vi "registerEvents.vi"(8 "error in (no error)":errorcluster, 10 "registeredEvents":string[][](array[string]), 11 "tcpServer in":refnum<class "TcpServer.lvclass">) -> (0 "error out":errorcluster, 3 "tcpServer out":refnum<class "TcpServer.lvclass">)   [LabVIEW 2018, in "TcpServer.lvclass"]
doc: "Inform the TCP Server which events are registered and allowed to be processed."
uses:
  TcpServer.lvclass
  TcpServer.lvclass/TcpServer.ctl
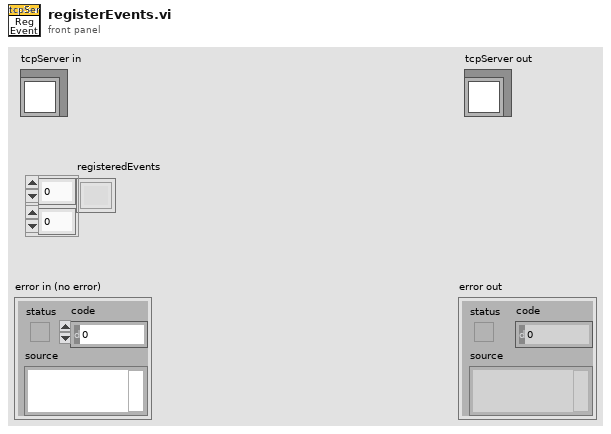
[diagram p1: front panel]
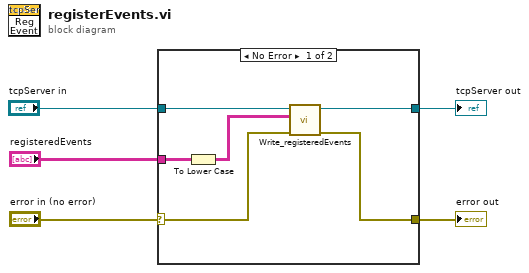
[diagram p0: block diagram]
diagram:
  n1 = case shown="No Error" "error in (no error)" {
    selector: "error in (no error)" -> [w8 w13]
    tunnel: [w7 w13] -> w4
    tunnel: [w10 w12] -> w2
    tunnel: "tcpServer in" -> [w11 w12]
    tunnel: "registeredEvents" -> [w9 _]
    frame No Error {
      n2 = To Lower Case(string=w9) -> (all lower case string=w6:string[][])
      n3 = call "Write_registeredEvents.vi"("error in (no error)"=w8, "registeredEvents"=w6, "TcpServer in"=w11) -> ("error out"=w7:errorcluster, "TcpServer out"=w10:refnum<class "TcpServer.lvclass">)  [unwired: 7 in]
    }
    frame Error {
    }
  }
  "error out" <- w4
  "tcpServer out" <- w2
